vi "BMU参数读取-Auto.vi"(7 "Socket":dbl, 8 "CAN端口":u16(ring), 9 "设备索引号":u16(ring), 10 "CAN卡类型":u32(ring)=21, 11 "从板号":u8=1) -> (3 "成功?":bool)   [LabVIEW 2013] (continued)
          event "读配置文件": Value Change {
            n3737 = event-data() -> ("NewVal"=w5416:bool)  [unwired: 6 out]
            n3738 = case shown="真" w5416 {
              tunnel: w5420 -> [w5422 w5427]
              tunnel: [w5422 w5426] -> w5419
              tunnel: w5418 -> [w5421 w5425]
              tunnel: [w5421 w5424] -> w5417
              frame False {
              }
              frame True {
                n3739 = Enqueue Element(queue=w5427, element="读配置文件", error in (no error)=w5425) -> (queue out=w5426:refnum<queue>, error out=w5424:errorcluster)  [unwired: 2 out]
                n3740 = call <vilib>:"Set Busy.vi"() -> ()  [unwired: 4 in, 8 out]
              }
            }
          }
          event "保存主板参数": Value Change {
            n3741 = event-data() -> ("NewVal"=w5428:bool)  [unwired: 6 out]
            n3742 = case shown="真" w5428 {
              tunnel: w5432 -> [w5434 w5439]
              tunnel: [w5434 w5438] -> w5431
              tunnel: w5430 -> [w5433 w5437]
              tunnel: [w5433 w5436] -> w5429
              frame False {
              }
              frame True {
                n3743 = Enqueue Element(queue=w5439, element="写配置文件", error in (no error)=w5437) -> (queue out=w5438:refnum<queue>, error out=w5436:errorcluster)  [unwired: 2 out]
              }
            }
          }
          event "继电器全开": Value Change {
            n3744 = event-data() -> ("NewVal"=w5440:bool)  [unwired: 6 out]
            n3745 = case shown="真" w5440 {
              tunnel: w5440 -> [_ w5443]
              frame False {
              }
              frame True {
                n3746 = stacked-sequence {
                  tunnel: w5443 -> [_ w5453 _]
                  frame #0 {
                    w5444 = FALSE ("清BUFF")
                    n3747 = local write "正级继电器"(w5444) -> ()
                    n3748 = local write "负级继电器"(w5444) -> ()
                    n3749 = local write "充电继电器"(w5444) -> ()
                    n3750 = local write "加热继电器"(w5444) -> ()
                    n3751 = local write "风机继电器"(w5444) -> ()
                    n3752 = local write "预充电继电器"(w5444) -> ()
                    n3753 = local write "继电器超时处理"(FALSE ("继电器超时处理")) -> ()
                    n3754 = local write "主从选择"(enum32{"主板", "从板"}."主板" ("主从选择")) -> ()
                    n3755 = local write "清BUFF"(FALSE ("清BUFF")) -> ()
                  }
                  frame #1 {
                    n3756 = case shown="真" w5453 {
                      selector: w5453 -> [_ w5468]
                      frame False {
                      }
                      frame True {
                        w5464 = 256.0 ("y")
                        w5455 = u32 1 ("命令序号")
                        w5454 = u8 192 ("命令")
                        n3757 = local read "动作保持时间"() -> (w5465:dbl)
                        n3758 = Quotient & Remainder(x=w5465, y=w5464) -> (x-y*floor(x/y)=w5457:dbl, floor(x/y)=w5461:dbl)
                        n3759 = Quotient & Remainder(x=w5461, y=w5464) -> (x-y*floor(x/y)=w5458:dbl, floor(x/y)=w5462:dbl)
                        n3760 = Quotient & Remainder(x=w5462, y=w5464) -> (x-y*floor(x/y)=w5459:dbl, floor(x/y)=w5463:dbl)
                        n3761 = local read "设备索引号"() -> (w5472:u16)
                        n3762 = local read "CAN卡类型"() -> (w5473:u32)
                        n3763 = local read "CAN端口"() -> (w5471:u16)
                        n3764 = Boolean To (0,1)(Boolean=w5468) -> (0, 1=w5466:i16)
                        n3765 = Quotient & Remainder(x=w5463, y=w5464) -> (x-y*floor(x/y)=w5460:dbl)  [unwired: 1 out]
                        n3766 = Build Array(i16 170 ("元素"), w5466, w5460, w5459, w5458, w5457, 0.0 ("元素")) -> (w5469:dbl[])
                        n3767 = call "多帧发送机制(EV05).vi"("can卡类型"=w5473, "设备索引号"=w5472, "CAN端口"=w5471, "命令"=w5454, "板号"=u8 0, "命令序号"=w5455, "输入数据"=w5469) -> ()  [unwired: 2 in, 11 out]
                        n3768 = local write "命令序号"(w5455) -> ()
                        n3769 = local write "命令"(w5454) -> ()
                      }
                    }
                    n3770 = local write "控制1"(TRUE ("控制1")) -> ()
                    n3771 = local write "写?"(FALSE ("写?")) -> ()
                    n3772 = local write "消除"(TRUE ("消除")) -> ()
                    n3773 = global write "EV05全局变量1.vi" "流控帧 2"(TRUE ("流控帧 2")) -> ()
                    n3774 = global write "EV05全局变量1.vi" "流控帧"(FALSE ("流控帧")) -> ()
                  }
                  frame #2 {
                    n3775 = flat-sequence {
                      tunnel: [w5475] -> w5474
                      tunnel: w5474 -> [w5482]
                      frame #0 {
                        n3776 = while {
                          tunnel: [w5476] -> w5475
                          i -> [w5480]
                          stop <- w5477 stop-if-true
                          n3777 = local read "继电器超时处理"() -> (w5476:bool)
                          n3778 = Greater Or Equal?(x=w5480, y=20) -> (x >= y?=w5478:bool)
                          n3779 = Wait Until Next ms Multiple(millisecond multiple=u32 100 ("毫秒倍数")) -> ()  [unwired: 1 out]
                          n3780 = Or(x=w5476, y=w5478) -> (x .or. y?=w5477:bool)
                        }
                      }
                      frame #1 {
                        n3781 = case shown="真" w5482 {
                          frame False {
                            n3782 = One Button Dialog(message="继电器处理超时" ("消息"), button name ("OK")="是" ("按钮名称（“确定”）")) -> ()  [unwired: 1 out]
                          }
                          frame True {
                            w5485 = TRUE ("清BUFF")
                            n3783 = local write "正级继电器"(w5485) -> ()
                            n3784 = local write "负级继电器"(w5485) -> ()
                            n3785 = local write "充电继电器"(w5485) -> ()
                            n3786 = local write "加热继电器"(w5485) -> ()
                            n3787 = local write "风机继电器"(w5485) -> ()
                            n3788 = local write "预充电继电器"(w5485) -> ()
                          }
                        }
                      }
                    }
                  }
                }
              }
            }
          }
          event "继电器全关": Value Change {
            n3789 = event-data() -> ("NewVal"=w5486:bool)  [unwired: 6 out]
            n3790 = case shown="真" w5486 {
              tunnel: w5486 -> [_ w5489]
              frame False {
              }
              frame True {
                n3791 = stacked-sequence {
                  tunnel: w5489 -> [_ w5499 _]
                  frame #0 {
                    w5490 = TRUE ("清BUFF")
                    n3792 = local write "正级继电器"(w5490) -> ()
                    n3793 = local write "负级继电器"(w5490) -> ()
                    n3794 = local write "充电继电器"(w5490) -> ()
                    n3795 = local write "加热继电器"(w5490) -> ()
                    n3796 = local write "风机继电器"(w5490) -> ()
                    n3797 = local write "预充电继电器"(w5490) -> ()
                    n3798 = local write "继电器超时处理"(FALSE ("继电器超时处理")) -> ()
                    n3799 = local write "主从选择"(enum32{"主板", "从板"}."主板" ("主从选择")) -> ()
                    n3800 = global write "EV05全局变量1.vi" "流控帧"(FALSE ("流控帧")) -> ()
                    n3801 = local write "清BUFF"(FALSE ("清BUFF")) -> ()
                  }
                  frame #1 {
                    n3802 = case shown="真" w5499 {
                      selector: w5499 -> [_ w5514]
                      frame False {
                      }
                      frame True {
                        w5510 = 256.0 ("y")
                        w5501 = u32 1 ("命令序号")
                        w5500 = u8 192 ("命令")
                        n3803 = local read "动作保持时间"() -> (w5511:dbl)
                        n3804 = Quotient & Remainder(x=w5511, y=w5510) -> (x-y*floor(x/y)=w5503:dbl, floor(x/y)=w5507:dbl)
                        n3805 = Quotient & Remainder(x=w5507, y=w5510) -> (x-y*floor(x/y)=w5504:dbl, floor(x/y)=w5508:dbl)
                        n3806 = Quotient & Remainder(x=w5508, y=w5510) -> (x-y*floor(x/y)=w5505:dbl, floor(x/y)=w5509:dbl)
                        n3807 = local read "设备索引号"() -> (w5518:u16)
                        n3808 = local read "CAN卡类型"() -> (w5519:u32)
                        n3809 = local read "CAN端口"() -> (w5517:u16)
                        n3810 = Boolean To (0,1)(Boolean=w5514) -> (0, 1=w5512:i16)
                        n3811 = Quotient & Remainder(x=w5509, y=w5510) -> (x-y*floor(x/y)=w5506:dbl)  [unwired: 1 out]
                        n3812 = Build Array(i16 85 ("元素"), w5512, w5506, w5505, w5504, w5503, 0.0 ("元素")) -> (w5515:dbl[])
                        n3813 = call "多帧发送机制(EV05).vi"("can卡类型"=w5519, "设备索引号"=w5518, "CAN端口"=w5517, "命令"=w5500, "板号"=u8 0, "命令序号"=w5501, "输入数据"=w5515) -> ()  [unwired: 2 in, 11 out]
                        n3814 = local write "命令序号"(w5501) -> ()
                        n3815 = local write "命令"(w5500) -> ()
                      }
                    }
                    n3816 = local write "控制1"(TRUE ("控制1")) -> ()
                    n3817 = local write "写?"(FALSE ("写?")) -> ()
                    n3818 = local write "消除"(TRUE ("消除")) -> ()
                    n3819 = global write "EV05全局变量1.vi" "流控帧 2"(TRUE ("流控帧 2")) -> ()
                  }
                  frame #2 {
                    n3820 = flat-sequence {
                      tunnel: [w5521] -> w5520
                      tunnel: w5520 -> [w5528]
                      frame #0 {
                        n3821 = while {
                          tunnel: [w5522] -> w5521
                          i -> [w5526]
                          stop <- w5523 stop-if-true
                          n3822 = local read "继电器超时处理"() -> (w5522:bool)
                          n3823 = Greater Or Equal?(x=w5526, y=20) -> (x >= y?=w5524:bool)
                          n3824 = Wait Until Next ms Multiple(millisecond multiple=u32 100 ("毫秒倍数")) -> ()  [unwired: 1 out]
                          n3825 = Or(x=w5522, y=w5524) -> (x .or. y?=w5523:bool)
                        }
                      }
                      frame #1 {
                        n3826 = case shown="真" w5528 {
                          frame False {
                            n3827 = One Button Dialog(message="继电器处理超时" ("消息"), button name ("OK")="是" ("按钮名称（“确定”）")) -> ()  [unwired: 1 out]
                          }
                          frame True {
                            w5531 = FALSE ("清BUFF")
                            n3828 = local write "正级继电器"(w5531) -> ()
                            n3829 = local write "负级继电器"(w5531) -> ()
                            n3830 = local write "充电继电器"(w5531) -> ()
                            n3831 = local write "加热继电器"(w5531) -> ()
                            n3832 = local write "风机继电器"(w5531) -> ()
                            n3833 = local write "预充电继电器"(w5531) -> ()
                          }
                        }
                      }
                    }
                  }
                }
              }
            }
          }
          event "控制按键全为开": Value Change {
            n3834 = event-data() -> ("NewVal"=w5532:bool)  [unwired: 6 out]
            n3835 = case shown="真" w5532 {
              frame False {
              }
              frame True {
                w5533 = TRUE ("正级继电器")
                n3836 = local write "加热继电器(从)"(w5533) -> ()
                n3837 = local write "风机继电器(从)"(w5533) -> ()
                n3838 = local write "DO1 2"(w5533) -> ()
                n3839 = local write "DO1"(w5533) -> ()
                n3840 = local write "DO2"(w5533) -> ()
                n3841 = local write "正级继电器"(w5533) -> ()
                n3842 = local write "负级继电器"(w5533) -> ()
                n3843 = local write "加热继电器"(w5533) -> ()
                n3844 = local write "预充电继电器"(w5533) -> ()
                n3845 = local write "充电继电器"(w5533) -> ()
                n3846 = local write "风机继电器"(w5533) -> ()
              }
            }
          }
          event "控制按键全为关": Value Change {
            n3847 = event-data() -> ("NewVal"=w5534:bool)  [unwired: 6 out]
            n3848 = case shown="真" w5534 {
              frame False {
              }
              frame True {
                w5535 = FALSE ("正级继电器")
                n3849 = local write "加热继电器(从)"(w5535) -> ()
                n3850 = local write "风机继电器(从)"(w5535) -> ()
                n3851 = local write "DO1 2"(w5535) -> ()
                n3852 = local write "DO1"(w5535) -> ()
                n3853 = local write "DO2"(w5535) -> ()
                n3854 = local write "正级继电器"(w5535) -> ()
                n3855 = local write "负级继电器"(w5535) -> ()
                n3856 = local write "加热继电器"(w5535) -> ()
                n3857 = local write "预充电继电器"(w5535) -> ()
                n3858 = local write "充电继电器"(w5535) -> ()
                n3859 = local write "风机继电器"(w5535) -> ()
              }
            }
          }
          event "正级继电器": Value Change {
            n3860 = event-data() -> ("NewVal"=w5536:bool)  [unwired: 6 out]
            n3861 = stacked-sequence {
              tunnel: w5536 -> [_ w5549 _]
              frame #0 {
                w5539 = FALSE ("清BUFF")
                n3862 = local write "继电器超时处理"(FALSE ("继电器超时处理")) -> ()
                n3863 = local write "主从选择"(enum32{"主板", "从板"}."主板" ("主从选择")) -> ()
                n3864 = local write "正级继电器 12"(w5539) -> ()
                n3865 = local write "清BUFF"(w5539) -> ()
              }
              frame #1 {
                n3866 = case shown="假" w5549 {
                  selector: w5549 -> [w5564 w5584]
                  tunnel: [w5563 w5583] -> w5548
                  tunnel: [w5551 w5571] -> w5543
                  frame False {
                    w5559 = 256.0 ("y")
                    w5551 = u32 1 ("命令序号")
                    w5563 = u8 192 ("命令")
                    n3867 = local read "动作保持时间"() -> (w5560:dbl)
                    n3868 = Quotient & Remainder(x=w5560, y=w5559) -> (x-y*floor(x/y)=w5552:dbl, floor(x/y)=w5556:dbl)
                    n3869 = Quotient & Remainder(x=w5556, y=w5559) -> (x-y*floor(x/y)=w5553:dbl, floor(x/y)=w5557:dbl)
                    n3870 = Quotient & Remainder(x=w5557, y=w5559) -> (x-y*floor(x/y)=w5554:dbl, floor(x/y)=w5558:dbl)
                    n3871 = local read "设备索引号"() -> (w5568:u16)
                    n3872 = local read "CAN卡类型"() -> (w5569:u32)
                    n3873 = local read "CAN端口"() -> (w5567:u16)
                    n3874 = Boolean To (0,1)(Boolean=w5564) -> (0, 1=w5561:i16)
                    n3875 = Quotient & Remainder(x=w5558, y=w5559) -> (x-y*floor(x/y)=w5555:dbl)  [unwired: 1 out]
                    n3876 = Build Array(i16 1 ("元素"), w5561, w5555, w5554, w5553, w5552, 0.0 ("元素")) -> (w5565:dbl[])
                    n3877 = call "多帧发送机制(EV05).vi"("can卡类型"=w5569, "设备索引号"=w5568, "CAN端口"=w5567, "命令"=w5563, "板号"=u8 0, "命令序号"=w5551, "输入数据"=w5565) -> ()  [unwired: 2 in, 11 out]
                  }
                  frame True {
                    w5579 = 256.0 ("y")
                    w5571 = u32 1 ("命令序号")
                    w5583 = u8 192 ("命令")
                    n3878 = local read "动作保持时间"() -> (w5580:dbl)
                    n3879 = Quotient & Remainder(x=w5580, y=w5579) -> (x-y*floor(x/y)=w5572:dbl, floor(x/y)=w5576:dbl)
                    n3880 = Quotient & Remainder(x=w5576, y=w5579) -> (x-y*floor(x/y)=w5573:dbl, floor(x/y)=w5577:dbl)
                    n3881 = Quotient & Remainder(x=w5577, y=w5579) -> (x-y*floor(x/y)=w5574:dbl, floor(x/y)=w5578:dbl)
                    n3882 = local read "设备索引号"() -> (w5588:u16)
                    n3883 = local read "CAN卡类型"() -> (w5589:u32)
                    n3884 = local read "CAN端口"() -> (w5587:u16)
                    n3885 = Boolean To (0,1)(Boolean=w5584) -> (0, 1=w5581:i16)
                    n3886 = Quotient & Remainder(x=w5578, y=w5579) -> (x-y*floor(x/y)=w5575:dbl)  [unwired: 1 out]
                    n3887 = Build Array(i16 1 ("元素"), w5581, w5575, w5574, w5573, w5572, 0.0 ("元素")) -> (w5585:dbl[])
                    n3888 = call "多帧发送机制(EV05).vi"("can卡类型"=w5589, "设备索引号"=w5588, "CAN端口"=w5587, "命令"=w5583, "板号"=u8 0, "命令序号"=w5571, "输入数据"=w5585) -> ()  [unwired: 2 in, 11 out]
                  }
                }
                n3889 = local write "命令序号"(w5543) -> ()
                n3890 = local write "命令"(w5548) -> ()
                n3891 = local write "控制1"(TRUE ("控制1")) -> ()
                n3892 = local write "写?"(FALSE ("写?")) -> ()
                n3893 = global write "EV05全局变量1.vi" "流控帧"(FALSE ("流控帧")) -> ()
                n3894 = local write "消除"(TRUE ("消除")) -> ()
                n3895 = global write "EV05全局变量1.vi" "流控帧 2"(TRUE ("流控帧 2")) -> ()
              }
              frame #2 {
                n3896 = flat-sequence {
                  tunnel: [w5591] -> w5590
                  tunnel: w5590 -> [w5598]
                  frame #0 {
                    n3897 = while {
                      tunnel: [w5592] -> w5591
                      i -> [w5596]
                      stop <- w5593 stop-if-true
                      n3898 = local read "继电器超时处理"() -> (w5592:bool)
                      n3899 = Greater Or Equal?(x=w5596, y=20) -> (x >= y?=w5594:bool)
                      n3900 = Wait Until Next ms Multiple(millisecond multiple=u32 100 ("毫秒倍数")) -> ()  [unwired: 1 out]
                      n3901 = Or(x=w5592, y=w5594) -> (x .or. y?=w5593:bool)
                    }
                  }
                  frame #1 {
                    n3902 = case shown="假" w5598 {
                      frame False {
                        n3903 = local read "正级继电器"() -> (w5600:bool)
                        n3904 = Not(x=w5600) -> (.not. x?=w5599:bool)
                        n3905 = local write "正级继电器"(w5599) -> ()
                        n3906 = One Button Dialog(message="继电器处理超时" ("消息"), button name ("OK")="是" ("按钮名称（“确定”）")) -> ()  [unwired: 1 out]
                      }
                      frame True {
                      }
                    }
                  }
                }
              }
            }
          }
          event "负级继电器": Value Change {
            n3907 = event-data() -> ("NewVal"=w5603:bool)  [unwired: 6 out]
            n3908 = stacked-sequence {
              tunnel: w5603 -> [_ w5616 _]
              frame #0 {
                w5606 = FALSE ("继电器超时处理")
                n3909 = local write "继电器超时处理"(w5606) -> ()
                n3910 = local write "正级继电器 2"(w5606) -> ()
                n3911 = local write "主从选择"(enum32{"主板", "从板"}."主板" ("主从选择")) -> ()
              }
              frame #1 {
                n3912 = case shown="假" w5616 {
                  selector: w5616 -> [w5630 w5650]
                  tunnel: [w5629 w5649] -> w5615
                  tunnel: [w5618 w5638] -> w5610
                  frame False {
                    w5626 = 256.0 ("y")
                    w5618 = u32 1 ("命令序号")
                    w5629 = u8 192 ("命令")
                    n3913 = local read "动作保持时间"() -> (w5627:dbl)
                    n3914 = Quotient & Remainder(x=w5627, y=w5626) -> (x-y*floor(x/y)=w5619:dbl, floor(x/y)=w5623:dbl)
                    n3915 = Quotient & Remainder(x=w5623, y=w5626) -> (x-y*floor(x/y)=w5620:dbl, floor(x/y)=w5624:dbl)
                    n3916 = Quotient & Remainder(x=w5624, y=w5626) -> (x-y*floor(x/y)=w5621:dbl, floor(x/y)=w5625:dbl)
                    n3917 = Quotient & Remainder(x=w5625, y=w5626) -> (x-y*floor(x/y)=w5622:dbl)  [unwired: 1 out]
                    n3918 = Boolean To (0,1)(Boolean=w5630) -> (0, 1=w5628:i16)
                    n3919 = local read "设备索引号"() -> (w5635:u16)
                    n3920 = local read "CAN卡类型"() -> (w5636:u32)
                    n3921 = local read "CAN端口"() -> (w5634:u16)
                    n3922 = Build Array(i16 2 ("元素"), w5628, w5622, w5621, w5620, w5619, 0.0 ("元素")) -> (w5632:dbl[])
                    n3923 = call "多帧发送机制(EV05).vi"("can卡类型"=w5636, "设备索引号"=w5635, "CAN端口"=w5634, "命令"=w5629, "板号"=u8 0, "命令序号"=w5618, "输入数据"=w5632) -> ()  [unwired: 2 in, 11 out]
                  }
                  frame True {
                    w5646 = 256.0 ("y")
                    w5638 = u32 1 ("命令序号")
                    w5649 = u8 192 ("命令")
                    n3924 = local read "动作保持时间"() -> (w5647:dbl)
                    n3925 = Quotient & Remainder(x=w5647, y=w5646) -> (x-y*floor(x/y)=w5639:dbl, floor(x/y)=w5643:dbl)
                    n3926 = Quotient & Remainder(x=w5643, y=w5646) -> (x-y*floor(x/y)=w5640:dbl, floor(x/y)=w5644:dbl)
                    n3927 = Quotient & Remainder(x=w5644, y=w5646) -> (x-y*floor(x/y)=w5641:dbl, floor(x/y)=w5645:dbl)
                    n3928 = Quotient & Remainder(x=w5645, y=w5646) -> (x-y*floor(x/y)=w5642:dbl)  [unwired: 1 out]
                    n3929 = Boolean To (0,1)(Boolean=w5650) -> (0, 1=w5648:i16)
                    n3930 = local read "设备索引号"() -> (w5655:u16)
                    n3931 = local read "CAN卡类型"() -> (w5656:u32)
                    n3932 = local read "CAN端口"() -> (w5654:u16)
                    n3933 = Build Array(i16 2 ("元素"), w5648, w5642, w5641, w5640, w5639, 0.0 ("元素")) -> (w5652:dbl[])
                    n3934 = call "多帧发送机制(EV05).vi"("can卡类型"=w5656, "设备索引号"=w5655, "CAN端口"=w5654, "命令"=w5649, "板号"=u8 0, "命令序号"=w5638, "输入数据"=w5652) -> ()  [unwired: 2 in, 11 out]
                  }
                }
                n3935 = local write "命令"(w5615) -> ()
                n3936 = local write "命令序号"(w5610) -> ()
                n3937 = local write "清BUFF"(FALSE ("清BUFF")) -> ()
                n3938 = global write "EV05全局变量1.vi" "流控帧"(FALSE ("流控帧")) -> ()
                n3939 = local write "控制1"(TRUE ("控制1")) -> ()
                n3940 = global write "EV05全局变量1.vi" "流控帧 2"(TRUE ("流控帧 2")) -> ()
                n3941 = local write "写?"(FALSE ("写?")) -> ()
                n3942 = local write "消除"(TRUE ("消除")) -> ()
              }
              frame #2 {
                n3943 = flat-sequence {
                  tunnel: [w5658] -> w5657
                  tunnel: w5657 -> [w5665]
                  frame #0 {
                    n3944 = while {
                      tunnel: [w5659] -> w5658
                      i -> [w5663]
                      stop <- w5660 stop-if-true
                      n3945 = local read "继电器超时处理"() -> (w5659:bool)
                      n3946 = Greater Or Equal?(x=w5663, y=20) -> (x >= y?=w5661:bool)
                      n3947 = Wait Until Next ms Multiple(millisecond multiple=u32 100 ("毫秒倍数")) -> ()  [unwired: 1 out]
                      n3948 = Or(x=w5659, y=w5661) -> (x .or. y?=w5660:bool)
                    }
                  }
                  frame #1 {
                    n3949 = case shown="假" w5665 {
                      frame False {
                        n3950 = local read "负级继电器"() -> (w5666:bool)
                        n3951 = Not(x=w5666) -> (.not. x?=w5667:bool)
                        n3952 = local write "负级继电器"(w5667) -> ()
                        n3953 = One Button Dialog(message="继电器处理超时" ("消息"), button name ("OK")="是" ("按钮名称（“确定”）")) -> ()  [unwired: 1 out]
                      }
                      frame True {
                      }
                    }
                  }
                }
              }
            }
          }
          event "预充电继电器": Value Change {
            n3954 = event-data() -> ("NewVal"=w5670:bool)  [unwired: 6 out]
            n3955 = stacked-sequence {
              tunnel: w5670 -> [_ w5683 _]
              frame #0 {
                w5674 = FALSE ("继电器超时处理")
                n3956 = local write "继电器超时处理"(w5674) -> ()
                n3957 = local write "正级继电器 3"(w5674) -> ()
                n3958 = global write "EV05全局变量1.vi" "流控帧"(FALSE ("流控帧")) -> ()
                n3959 = local write "主从选择"(enum32{"主板", "从板"}."主板" ("主从选择")) -> ()
              }
              frame #1 {
                n3960 = case shown="假" w5683 {
                  selector: w5683 -> [w5697 w5717]
                  tunnel: [w5696 w5716] -> w5682
                  tunnel: [w5685 w5705] -> w5677
                  frame False {
                    w5693 = 256.0 ("y")
                    w5685 = u32 1 ("命令序号")
                    w5696 = u8 192 ("命令")
                    n3961 = local read "动作保持时间"() -> (w5694:dbl)
                    n3962 = Quotient & Remainder(x=w5694, y=w5693) -> (x-y*floor(x/y)=w5686:dbl, floor(x/y)=w5690:dbl)
                    n3963 = Quotient & Remainder(x=w5690, y=w5693) -> (x-y*floor(x/y)=w5687:dbl, floor(x/y)=w5691:dbl)
                    n3964 = Quotient & Remainder(x=w5691, y=w5693) -> (x-y*floor(x/y)=w5688:dbl, floor(x/y)=w5692:dbl)
                    n3965 = Quotient & Remainder(x=w5692, y=w5693) -> (x-y*floor(x/y)=w5689:dbl)  [unwired: 1 out]
                    n3966 = Boolean To (0,1)(Boolean=w5697) -> (0, 1=w5695:i16)
                    n3967 = local read "设备索引号"() -> (w5702:u16)
                    n3968 = local read "CAN卡类型"() -> (w5703:u32)
                    n3969 = local read "CAN端口"() -> (w5701:u16)
                    n3970 = Build Array(i16 3 ("元素"), w5695, w5689, w5688, w5687, w5686, 0.0 ("元素")) -> (w5699:dbl[])
                    n3971 = call "多帧发送机制(EV05).vi"("can卡类型"=w5703, "设备索引号"=w5702, "CAN端口"=w5701, "命令"=w5696, "板号"=u8 0, "命令序号"=w5685, "输入数据"=w5699) -> ()  [unwired: 2 in, 11 out]
                  }
                  frame True {
                    w5713 = 256.0 ("y")
                    w5705 = u32 1 ("命令序号")
                    w5716 = u8 192 ("命令")
                    n3972 = local read "动作保持时间"() -> (w5714:dbl)
                    n3973 = Quotient & Remainder(x=w5714, y=w5713) -> (x-y*floor(x/y)=w5706:dbl, floor(x/y)=w5710:dbl)
                    n3974 = Quotient & Remainder(x=w5710, y=w5713) -> (x-y*floor(x/y)=w5707:dbl, floor(x/y)=w5711:dbl)
                    n3975 = Quotient & Remainder(x=w5711, y=w5713) -> (x-y*floor(x/y)=w5708:dbl, floor(x/y)=w5712:dbl)
                    n3976 = Quotient & Remainder(x=w5712, y=w5713) -> (x-y*floor(x/y)=w5709:dbl)  [unwired: 1 out]
                    n3977 = Boolean To (0,1)(Boolean=w5717) -> (0, 1=w5715:i16)
                    n3978 = local read "设备索引号"() -> (w5722:u16)
                    n3979 = local read "CAN卡类型"() -> (w5723:u32)
                    n3980 = local read "CAN端口"() -> (w5721:u16)
                    n3981 = Build Array(i16 3 ("元素"), w5715, w5709, w5708, w5707, w5706, 0.0 ("元素")) -> (w5719:dbl[])
                    n3982 = call "多帧发送机制(EV05).vi"("can卡类型"=w5723, "设备索引号"=w5722, "CAN端口"=w5721, "命令"=w5716, "板号"=u8 0, "命令序号"=w5705, "输入数据"=w5719) -> ()  [unwired: 2 in, 11 out]
                  }
                }
                n3983 = local write "命令序号"(w5677) -> ()
                n3984 = local write "清BUFF"(FALSE ("清BUFF")) -> ()
                n3985 = local write "控制1"(TRUE ("控制1")) -> ()
                n3986 = global write "EV05全局变量1.vi" "流控帧 2"(TRUE ("流控帧 2")) -> ()
                n3987 = local write "消除"(TRUE ("消除")) -> ()
                n3988 = local write "命令"(w5682) -> ()
                n3989 = local write "写?"(FALSE ("写?")) -> ()
              }
              frame #2 {
                n3990 = flat-sequence {
                  tunnel: [w5725] -> w5724
                  tunnel: w5724 -> [w5732]
                  frame #0 {
                    n3991 = while {
                      tunnel: [w5726] -> w5725
                      i -> [w5730]
                      stop <- w5727 stop-if-true
                      n3992 = local read "继电器超时处理"() -> (w5726:bool)
                      n3993 = Greater Or Equal?(x=w5730, y=20) -> (x >= y?=w5728:bool)
                      n3994 = Wait Until Next ms Multiple(millisecond multiple=u32 100 ("毫秒倍数")) -> ()  [unwired: 1 out]
                      n3995 = Or(x=w5726, y=w5728) -> (x .or. y?=w5727:bool)
                    }
                  }
                  frame #1 {
                    n3996 = case shown="假" w5732 {
                      frame False {
                        n3997 = local read "预充电继电器"() -> (w5733:bool)
                        n3998 = Not(x=w5733) -> (.not. x?=w5734:bool)
                        n3999 = local write "预充电继电器"(w5734) -> ()
                        n4000 = One Button Dialog(message="继电器处理超时" ("消息"), button name ("OK")="是" ("按钮名称（“确定”）")) -> ()  [unwired: 1 out]
                      }
                      frame True {
                      }
                    }
                  }
                }
              }
            }
          }
          event "加热继电器": Value Change {
            n4001 = event-data() -> ("NewVal"=w5737:bool)  [unwired: 6 out]
            n4002 = stacked-sequence {
              tunnel: w5737 -> [_ w5750 _]
              frame #0 {
                w5741 = FALSE ("继电器超时处理")
                n4003 = local write "继电器超时处理"(w5741) -> ()
                n4004 = local write "正级继电器 5"(w5741) -> ()
                n4005 = global write "EV05全局变量1.vi" "流控帧"(FALSE ("流控帧")) -> ()
                n4006 = local write "主从选择"(enum32{"主板", "从板"}."主板" ("主从选择")) -> ()
              }
              frame #1 {
                n4007 = case shown="假" w5750 {
                  selector: w5750 -> [w5764 w5784]
                  tunnel: [w5763 w5783] -> w5749
                  tunnel: [w5752 w5772] -> w5744
                  frame False {
                    w5760 = 256.0 ("y")
                    w5752 = u32 1 ("命令序号")
                    w5763 = u8 192 ("命令")
                    n4008 = local read "动作保持时间"() -> (w5761:dbl)
                    n4009 = Quotient & Remainder(x=w5761, y=w5760) -> (x-y*floor(x/y)=w5753:dbl, floor(x/y)=w5757:dbl)
                    n4010 = Quotient & Remainder(x=w5757, y=w5760) -> (x-y*floor(x/y)=w5754:dbl, floor(x/y)=w5758:dbl)
                    n4011 = Quotient & Remainder(x=w5758, y=w5760) -> (x-y*floor(x/y)=w5755:dbl, floor(x/y)=w5759:dbl)
                    n4012 = Quotient & Remainder(x=w5759, y=w5760) -> (x-y*floor(x/y)=w5756:dbl)  [unwired: 1 out]
                    n4013 = Boolean To (0,1)(Boolean=w5764) -> (0, 1=w5762:i16)
                    n4014 = local read "设备索引号"() -> (w5769:u16)
                    n4015 = local read "CAN卡类型"() -> (w5770:u32)
                    n4016 = local read "CAN端口"() -> (w5768:u16)
                    n4017 = Build Array(i16 4 ("元素"), w5762, w5756, w5755, w5754, w5753, 0.0 ("元素")) -> (w5766:dbl[])
                    n4018 = call "多帧发送机制(EV05).vi"("can卡类型"=w5770, "设备索引号"=w5769, "CAN端口"=w5768, "命令"=w5763, "板号"=u8 0, "命令序号"=w5752, "输入数据"=w5766) -> ()  [unwired: 2 in, 11 out]
                  }
                  frame True {
                    w5780 = 256.0 ("y")
                    w5772 = u32 1 ("命令序号")
                    w5783 = u8 192 ("命令")
                    n4019 = local read "动作保持时间"() -> (w5781:dbl)
                    n4020 = Quotient & Remainder(x=w5781, y=w5780) -> (x-y*floor(x/y)=w5773:dbl, floor(x/y)=w5777:dbl)
                    n4021 = Quotient & Remainder(x=w5777, y=w5780) -> (x-y*floor(x/y)=w5774:dbl, floor(x/y)=w5778:dbl)
                    n4022 = Quotient & Remainder(x=w5778, y=w5780) -> (x-y*floor(x/y)=w5775:dbl, floor(x/y)=w5779:dbl)
                    n4023 = Quotient & Remainder(x=w5779, y=w5780) -> (x-y*floor(x/y)=w5776:dbl)  [unwired: 1 out]
                    n4024 = Boolean To (0,1)(Boolean=w5784) -> (0, 1=w5782:i16)
                    n4025 = local read "设备索引号"() -> (w5789:u16)
                    n4026 = local read "CAN卡类型"() -> (w5790:u32)
                    n4027 = local read "CAN端口"() -> (w5788:u16)
                    n4028 = Build Array(i16 4 ("元素"), w5782, w5776, w5775, w5774, w5773, 0.0 ("元素")) -> (w5786:dbl[])
                    n4029 = call "多帧发送机制(EV05).vi"("can卡类型"=w5790, "设备索引号"=w5789, "CAN端口"=w5788, "命令"=w5783, "板号"=u8 0, "命令序号"=w5772, "输入数据"=w5786) -> ()  [unwired: 2 in, 11 out]
                  }
                }
                n4030 = local write "命令序号"(w5744) -> ()
                n4031 = local write "清BUFF"(FALSE ("清BUFF")) -> ()
                n4032 = local write "命令"(w5749) -> ()
                n4033 = local write "控制1"(TRUE ("控制1")) -> ()
                n4034 = local write "写?"(FALSE ("写?")) -> ()
                n4035 = global write "EV05全局变量1.vi" "流控帧 2"(TRUE ("流控帧 2")) -> ()
                n4036 = local write "消除"(TRUE ("消除")) -> ()
              }
              frame #2 {
                n4037 = flat-sequence {
                  tunnel: [w5792] -> w5791
                  tunnel: w5791 -> [w5799]
                  frame #0 {
                    n4038 = while {
                      tunnel: [w5793] -> w5792
                      i -> [w5797]
                      stop <- w5794 stop-if-true
                      n4039 = local read "继电器超时处理"() -> (w5793:bool)
                      n4040 = Greater Or Equal?(x=w5797, y=20) -> (x >= y?=w5795:bool)
                      n4041 = Wait Until Next ms Multiple(millisecond multiple=u32 100 ("毫秒倍数")) -> ()  [unwired: 1 out]
                      n4042 = Or(x=w5793, y=w5795) -> (x .or. y?=w5794:bool)
                    }
                  }
                  frame #1 {
                    n4043 = case shown="假" w5799 {
                      frame False {
                        n4044 = local read "加热继电器"() -> (w5800:bool)
                        n4045 = Not(x=w5800) -> (.not. x?=w5801:bool)
                        n4046 = local write "加热继电器"(w5801) -> ()
                        n4047 = One Button Dialog(message="继电器处理超时" ("消息"), button name ("OK")="是" ("按钮名称（“确定”）")) -> ()  [unwired: 1 out]
                      }
                      frame True {
                      }
                    }
                  }
                }
              }
            }
          }
          event "充电继电器": Value Change {
            n4048 = event-data() -> ("NewVal"=w5804:bool)  [unwired: 6 out]
            n4049 = stacked-sequence {
              tunnel: w5804 -> [_ w5817 _]
              frame #0 {
                w5808 = FALSE ("继电器超时处理")
                n4050 = local write "主从选择"(enum32{"主板", "从板"}."主板" ("主从选择")) -> ()
                n4051 = global write "EV05全局变量1.vi" "流控帧"(FALSE ("流控帧")) -> ()
                n4052 = local write "继电器超时处理"(w5808) -> ()
                n4053 = local write "正级继电器 4"(w5808) -> ()
              }
              frame #1 {
                n4054 = case shown="假" w5817 {
                  selector: w5817 -> [w5831 w5851]
                  tunnel: [w5830 w5850] -> w5816
                  tunnel: [w5819 w5839] -> w5811
                  frame False {
                    w5827 = 256.0 ("y")
                    w5819 = u32 1 ("命令序号")
                    w5830 = u8 192 ("命令")
                    n4055 = local read "动作保持时间"() -> (w5828:dbl)
                    n4056 = Quotient & Remainder(x=w5828, y=w5827) -> (x-y*floor(x/y)=w5820:dbl, floor(x/y)=w5824:dbl)
                    n4057 = Quotient & Remainder(x=w5824, y=w5827) -> (x-y*floor(x/y)=w5821:dbl, floor(x/y)=w5825:dbl)
                    n4058 = Quotient & Remainder(x=w5825, y=w5827) -> (x-y*floor(x/y)=w5822:dbl, floor(x/y)=w5826:dbl)
                    n4059 = Quotient & Remainder(x=w5826, y=w5827) -> (x-y*floor(x/y)=w5823:dbl)  [unwired: 1 out]
                    n4060 = Boolean To (0,1)(Boolean=w5831) -> (0, 1=w5829:i16)
                    n4061 = local read "设备索引号"() -> (w5836:u16)
                    n4062 = local read "CAN卡类型"() -> (w5837:u32)
                    n4063 = local read "CAN端口"() -> (w5835:u16)
                    n4064 = Build Array(i16 5 ("元素"), w5829, w5823, w5822, w5821, w5820, 0.0 ("元素")) -> (w5833:dbl[])
                    n4065 = call "多帧发送机制(EV05).vi"("can卡类型"=w5837, "设备索引号"=w5836, "CAN端口"=w5835, "命令"=w5830, "板号"=u8 0, "命令序号"=w5819, "输入数据"=w5833) -> ()  [unwired: 2 in, 11 out]
                  }
                  frame True {
                    w5847 = 256.0 ("y")
                    w5839 = u32 1 ("命令序号")
                    w5850 = u8 192 ("命令")
                    n4066 = local read "动作保持时间"() -> (w5848:dbl)
                    n4067 = Quotient & Remainder(x=w5848, y=w5847) -> (x-y*floor(x/y)=w5840:dbl, floor(x/y)=w5844:dbl)
                    n4068 = Quotient & Remainder(x=w5844, y=w5847) -> (x-y*floor(x/y)=w5841:dbl, floor(x/y)=w5845:dbl)
                    n4069 = Quotient & Remainder(x=w5845, y=w5847) -> (x-y*floor(x/y)=w5842:dbl, floor(x/y)=w5846:dbl)
                    n4070 = Quotient & Remainder(x=w5846, y=w5847) -> (x-y*floor(x/y)=w5843:dbl)  [unwired: 1 out]
                    n4071 = Boolean To (0,1)(Boolean=w5851) -> (0, 1=w5849:i16)
                    n4072 = local read "设备索引号"() -> (w5856:u16)
                    n4073 = local read "CAN卡类型"() -> (w5857:u32)
                    n4074 = local read "CAN端口"() -> (w5855:u16)
                    n4075 = Build Array(i16 5 ("元素"), w5849, w5843, w5842, w5841, w5840, 0.0 ("元素")) -> (w5853:dbl[])
                    n4076 = call "多帧发送机制(EV05).vi"("can卡类型"=w5857, "设备索引号"=w5856, "CAN端口"=w5855, "命令"=w5850, "板号"=u8 0, "命令序号"=w5839, "输入数据"=w5853) -> ()  [unwired: 2 in, 11 out]
                  }
                }
                n4077 = local write "命令序号"(w5811) -> ()
                n4078 = local write "命令"(w5816) -> ()
                n4079 = local write "清BUFF"(FALSE ("清BUFF")) -> ()
                n4080 = local write "控制1"(TRUE ("控制1")) -> ()
                n4081 = global write "EV05全局变量1.vi" "流控帧 2"(TRUE ("流控帧 2")) -> ()
                n4082 = local write "写?"(FALSE ("写?")) -> ()
                n4083 = local write "消除"(TRUE ("消除")) -> ()
              }
              frame #2 {
                n4084 = flat-sequence {
                  tunnel: [w5859] -> w5858
                  tunnel: w5858 -> [w5866]
                  frame #0 {
                    n4085 = while {
                      tunnel: [w5860] -> w5859
                      i -> [w5864]
                      stop <- w5861 stop-if-true
                      n4086 = local read "继电器超时处理"() -> (w5860:bool)
                      n4087 = Greater Or Equal?(x=w5864, y=20) -> (x >= y?=w5862:bool)
                      n4088 = Wait Until Next ms Multiple(millisecond multiple=u32 100 ("毫秒倍数")) -> ()  [unwired: 1 out]
                      n4089 = Or(x=w5860, y=w5862) -> (x .or. y?=w5861:bool)
                    }
                  }
                  frame #1 {
                    n4090 = case shown="假" w5866 {
                      frame False {
                        n4091 = local read "充电继电器"() -> (w5867:bool)
                        n4092 = Not(x=w5867) -> (.not. x?=w5868:bool)
                        n4093 = local write "充电继电器"(w5868) -> ()
                        n4094 = One Button Dialog(message="继电器处理超时" ("消息"), button name ("OK")="是" ("按钮名称（“确定”）")) -> ()  [unwired: 1 out]
                      }
                      frame True {
                      }
                    }
                  }
                }
              }
            }
          }
          event "风机继电器": Value Change {
            n4095 = event-data() -> ("NewVal"=w5871:bool)  [unwired: 6 out]
            n4096 = stacked-sequence {
              tunnel: w5871 -> [_ w5884 _]
              frame #0 {
                w5875 = FALSE ("继电器超时处理")
                n4097 = local write "继电器超时处理"(w5875) -> ()
                n4098 = local write "正级继电器 6"(w5875) -> ()
                n4099 = global write "EV05全局变量1.vi" "流控帧"(FALSE ("流控帧")) -> ()
                n4100 = local write "主从选择"(enum32{"主板", "从板"}."主板" ("主从选择")) -> ()
              }
              frame #1 {
                n4101 = case shown="真" w5884 {
                  selector: w5884 -> [w5898 w5918]
                  tunnel: [w5897 w5917] -> w5883
                  tunnel: [w5886 w5906] -> w5878
                  frame True {
                    w5894 = 256.0 ("y")
                    w5886 = u32 1 ("命令序号")
                    w5897 = u8 192 ("命令")
                    n4102 = local read "动作保持时间"() -> (w5895:dbl)
                    n4103 = Quotient & Remainder(x=w5895, y=w5894) -> (x-y*floor(x/y)=w5887:dbl, floor(x/y)=w5891:dbl)
                    n4104 = Quotient & Remainder(x=w5891, y=w5894) -> (x-y*floor(x/y)=w5888:dbl, floor(x/y)=w5892:dbl)
                    n4105 = Quotient & Remainder(x=w5892, y=w5894) -> (x-y*floor(x/y)=w5889:dbl, floor(x/y)=w5893:dbl)
                    n4106 = Boolean To (0,1)(Boolean=w5898) -> (0, 1=w5896:i16)
                    n4107 = local read "设备索引号"() -> (w5903:u16)
                    n4108 = local read "CAN卡类型"() -> (w5904:u32)
                    n4109 = Quotient & Remainder(x=w5893, y=w5894) -> (x-y*floor(x/y)=w5890:dbl)  [unwired: 1 out]
                    n4110 = local read "CAN端口"() -> (w5902:u16)
                    n4111 = Build Array(i16 6 ("元素"), w5896, w5890, w5889, w5888, w5887, 0.0 ("元素")) -> (w5900:dbl[])
                    n4112 = call "多帧发送机制(EV05).vi"("can卡类型"=w5904, "设备索引号"=w5903, "CAN端口"=w5902, "命令"=w5897, "板号"=u8 0, "命令序号"=w5886, "输入数据"=w5900) -> ()  [unwired: 2 in, 11 out]
                  }
                  frame False {
                    w5914 = 256.0 ("y")
                    w5906 = u32 1 ("命令序号")
                    w5917 = u8 192 ("命令")
                    n4113 = local read "动作保持时间"() -> (w5915:dbl)
                    n4114 = Quotient & Remainder(x=w5915, y=w5914) -> (x-y*floor(x/y)=w5907:dbl, floor(x/y)=w5911:dbl)
                    n4115 = Quotient & Remainder(x=w5911, y=w5914) -> (x-y*floor(x/y)=w5908:dbl, floor(x/y)=w5912:dbl)
                    n4116 = Quotient & Remainder(x=w5912, y=w5914) -> (x-y*floor(x/y)=w5909:dbl, floor(x/y)=w5913:dbl)
                    n4117 = Boolean To (0,1)(Boolean=w5918) -> (0, 1=w5916:i16)
                    n4118 = local read "设备索引号"() -> (w5923:u16)
                    n4119 = local read "CAN卡类型"() -> (w5924:u32)
                    n4120 = Quotient & Remainder(x=w5913, y=w5914) -> (x-y*floor(x/y)=w5910:dbl)  [unwired: 1 out]
                    n4121 = local read "CAN端口"() -> (w5922:u16)
                    n4122 = Build Array(i16 6 ("元素"), w5916, w5910, w5909, w5908, w5907, 0.0 ("元素")) -> (w5920:dbl[])
                    n4123 = call "多帧发送机制(EV05).vi"("can卡类型"=w5924, "设备索引号"=w5923, "CAN端口"=w5922, "命令"=w5917, "板号"=u8 0, "命令序号"=w5906, "输入数据"=w5920) -> ()  [unwired: 2 in, 11 out]
                  }
                }
                n4124 = local write "命令序号"(w5878) -> ()
                n4125 = local write "命令"(w5883) -> ()
                n4126 = local write "清BUFF"(FALSE ("清BUFF")) -> ()
                n4127 = local write "控制1"(TRUE ("控制1")) -> ()
                n4128 = global write "EV05全局变量1.vi" "流控帧 2"(TRUE ("流控帧 2")) -> ()
                n4129 = local write "写?"(FALSE ("写?")) -> ()
                n4130 = local write "消除"(TRUE ("消除")) -> ()
              }
              frame #2 {
                n4131 = flat-sequence {
                  tunnel: [w5926] -> w5925
                  tunnel: w5925 -> [w5933]
                  frame #0 {
                    n4132 = while {
                      tunnel: [w5927] -> w5926
                      i -> [w5931]
                      stop <- w5928 stop-if-true
                      n4133 = local read "继电器超时处理"() -> (w5927:bool)
                      n4134 = Greater Or Equal?(x=w5931, y=20) -> (x >= y?=w5929:bool)
                      n4135 = Wait Until Next ms Multiple(millisecond multiple=u32 100 ("毫秒倍数")) -> ()  [unwired: 1 out]
                      n4136 = Or(x=w5927, y=w5929) -> (x .or. y?=w5928:bool)
                    }
                  }
                  frame #1 {
                    n4137 = case shown="假" w5933 {
                      frame False {
                        n4138 = local read "风机继电器"() -> (w5934:bool)
                        n4139 = Not(x=w5934) -> (.not. x?=w5935:bool)
                        n4140 = local write "风机继电器"(w5935) -> ()
                        n4141 = One Button Dialog(message="继电器处理超时" ("消息"), button name ("OK")="是" ("按钮名称（“确定”）")) -> ()  [unwired: 1 out]
                      }
                      frame True {
                      }
                    }
                  }
                }
              }
            }
          }
          event "加热继电器(从)": Value Change {
            n4142 = event-data() -> ("NewVal"=w5938:bool)  [unwired: 6 out]
            n4143 = stacked-sequence {
              tunnel: w5938 -> [_ w5952 _]
              frame #0 {
                w5942 = FALSE ("继电器超时处理")
                n4144 = local write "正级继电器 7"(w5942) -> ()
                n4145 = local write "继电器超时处理"(w5942) -> ()
                n4146 = global write "EV05全局变量1.vi" "流控帧"(FALSE ("流控帧")) -> ()
                n4147 = local write "主从选择"(enum32{"主板", "从板"}."从板" ("主从选择")) -> ()
              }
              frame #1 {
                n4148 = case shown="真" w5952 {
                  selector: w5952 -> [w5967 w5987]
                  tunnel: [w5966 w5986] -> w5951
                  tunnel: [w5965 w5985] -> w5945
                  tunnel: [w5954 w5974] -> w5946
                  frame True {
                    w5962 = 256.0 ("y")
                    w5954 = u32 1 ("命令序号")
                    w5966 = u8 192 ("命令")
                    n4149 = local read "动作保持时间"() -> (w5963:dbl)
                    n4150 = Quotient & Remainder(x=w5963, y=w5962) -> (x-y*floor(x/y)=w5955:dbl, floor(x/y)=w5959:dbl)
                    n4151 = Quotient & Remainder(x=w5959, y=w5962) -> (x-y*floor(x/y)=w5956:dbl, floor(x/y)=w5960:dbl)
                    n4152 = Quotient & Remainder(x=w5960, y=w5962) -> (x-y*floor(x/y)=w5957:dbl, floor(x/y)=w5961:dbl)
                    n4153 = Quotient & Remainder(x=w5961, y=w5962) -> (x-y*floor(x/y)=w5958:dbl)  [unwired: 1 out]
                    n4154 = Boolean To (0,1)(Boolean=w5967) -> (0, 1=w5964:i16)
                    n4155 = local read "设备索引号"() -> (w5971:u16)
                    n4156 = local read "CAN卡类型"() -> (w5972:u32)
                    n4157 = local read "从板板号"() -> (w5965:u8)
                    n4158 = local read "CAN端口"() -> (w5970:u16)
                    n4159 = Build Array(i16 7 ("元素"), w5964, w5958, w5957, w5956, w5955, 0.0 ("元素")) -> (w5969:dbl[])
                    n4160 = call "多帧发送机制(EV05).vi"("can卡类型"=w5972, "设备索引号"=w5971, "CAN端口"=w5970, "命令"=w5966, "板号"=w5965, "命令序号"=w5954, "输入数据"=w5969) -> ()  [unwired: 2 in, 11 out]
                  }
                  frame False {
                    w5982 = 256.0 ("y")
                    w5974 = u32 1 ("命令序号")
                    w5986 = u8 192 ("命令")
                    n4161 = local read "动作保持时间"() -> (w5983:dbl)
                    n4162 = Quotient & Remainder(x=w5983, y=w5982) -> (x-y*floor(x/y)=w5975:dbl, floor(x/y)=w5979:dbl)
                    n4163 = Quotient & Remainder(x=w5979, y=w5982) -> (x-y*floor(x/y)=w5976:dbl, floor(x/y)=w5980:dbl)
                    n4164 = Quotient & Remainder(x=w5980, y=w5982) -> (x-y*floor(x/y)=w5977:dbl, floor(x/y)=w5981:dbl)
                    n4165 = Quotient & Remainder(x=w5981, y=w5982) -> (x-y*floor(x/y)=w5978:dbl)  [unwired: 1 out]
                    n4166 = Boolean To (0,1)(Boolean=w5987) -> (0, 1=w5984:i16)
                    n4167 = local read "设备索引号"() -> (w5991:u16)
                    n4168 = local read "CAN卡类型"() -> (w5992:u32)
                    n4169 = local read "从板板号"() -> (w5985:u8)
                    n4170 = local read "CAN端口"() -> (w5990:u16)
                    n4171 = Build Array(i16 7 ("元素"), w5984, w5978, w5977, w5976, w5975, 0.0 ("元素")) -> (w5989:dbl[])
                    n4172 = call "多帧发送机制(EV05).vi"("can卡类型"=w5992, "设备索引号"=w5991, "CAN端口"=w5990, "命令"=w5986, "板号"=w5985, "命令序号"=w5974, "输入数据"=w5989) -> ()  [unwired: 2 in, 11 out]
                  }
                }
                n4173 = local write "从板板号"(w5945) -> ()
                n4174 = local write "命令序号"(w5946) -> ()
                n4175 = local write "命令"(w5951) -> ()
                n4176 = local write "清BUFF"(FALSE ("清BUFF")) -> ()
                n4177 = local write "写?"(FALSE ("写?")) -> ()
                n4178 = local write "控制1"(TRUE ("控制1")) -> ()
                n4179 = global write "EV05全局变量1.vi" "流控帧 2"(TRUE ("流控帧 2")) -> ()
                n4180 = local write "消除"(TRUE ("消除")) -> ()
              }
              frame #2 {
                n4181 = flat-sequence {
                  tunnel: [w5994] -> w5993
                  tunnel: w5993 -> [w6001]
                  frame #0 {
                    n4182 = while {
                      tunnel: [w5995] -> w5994
                      i -> [w5999]
                      stop <- w5996 stop-if-true
                      n4183 = local read "继电器超时处理"() -> (w5995:bool)
                      n4184 = Greater Or Equal?(x=w5999, y=20) -> (x >= y?=w5997:bool)
                      n4185 = Wait Until Next ms Multiple(millisecond multiple=u32 100 ("毫秒倍数")) -> ()  [unwired: 1 out]
                      n4186 = Or(x=w5995, y=w5997) -> (x .or. y?=w5996:bool)
                    }
                  }
                  frame #1 {
                    n4187 = case shown="假" w6001 {
                      frame False {
                        n4188 = local read "加热继电器(从)"() -> (w6003:bool)
                        n4189 = Not(x=w6003) -> (.not. x?=w6002:bool)
                        n4190 = local write "加热继电器(从)"(w6002) -> ()
                        n4191 = One Button Dialog(message="继电器处理超时" ("消息"), button name ("OK")="是" ("按钮名称（“确定”）")) -> ()  [unwired: 1 out]
                      }
                      frame True {
                      }
                    }
                  }
                }
              }
            }
          }
          event "风机继电器(从)": Value Change {
            n4192 = event-data() -> ("NewVal"=w6006:bool)  [unwired: 6 out]
            n4193 = stacked-sequence {
              tunnel: w6006 -> [_ w6020 _]
              frame #0 {
                w6010 = FALSE ("继电器超时处理")
                n4194 = local write "继电器超时处理"(w6010) -> ()
                n4195 = local write "正级继电器 8"(w6010) -> ()
                n4196 = global write "EV05全局变量1.vi" "流控帧"(FALSE ("流控帧")) -> ()
                n4197 = local write "主从选择"(enum32{"主板", "从板"}."从板" ("主从选择")) -> ()
              }
              frame #1 {
                n4198 = case shown="假" w6020 {
                  selector: w6020 -> [w6035 w6055]
                  tunnel: [w6034 w6054] -> w6019
                  tunnel: [w6033 w6053] -> w6013
                  tunnel: [w6022 w6042] -> w6014
                  frame False {
                    w6030 = 256.0 ("y")
                    w6022 = u32 1 ("命令序号")
                    w6034 = u8 192 ("命令")
                    n4199 = local read "动作保持时间"() -> (w6031:dbl)
                    n4200 = Quotient & Remainder(x=w6031, y=w6030) -> (x-y*floor(x/y)=w6023:dbl, floor(x/y)=w6027:dbl)
                    n4201 = Quotient & Remainder(x=w6027, y=w6030) -> (x-y*floor(x/y)=w6024:dbl, floor(x/y)=w6028:dbl)
                    n4202 = Quotient & Remainder(x=w6028, y=w6030) -> (x-y*floor(x/y)=w6025:dbl, floor(x/y)=w6029:dbl)
                    n4203 = Quotient & Remainder(x=w6029, y=w6030) -> (x-y*floor(x/y)=w6026:dbl)  [unwired: 1 out]
                    n4204 = local read "设备索引号"() -> (w6039:u16)
                    n4205 = local read "CAN卡类型"() -> (w6040:u32)
                    n4206 = local read "从板板号"() -> (w6033:u8)
                    n4207 = Boolean To (0,1)(Boolean=w6035) -> (0, 1=w6032:i16)
                    n4208 = local read "CAN端口"() -> (w6038:u16)
                    n4209 = Build Array(i16 8 ("元素"), w6032, w6026, w6025, w6024, w6023, 0.0 ("元素")) -> (w6037:dbl[])
                    n4210 = call "多帧发送机制(EV05).vi"("can卡类型"=w6040, "设备索引号"=w6039, "CAN端口"=w6038, "命令"=w6034, "板号"=w6033, "命令序号"=w6022, "输入数据"=w6037) -> ()  [unwired: 2 in, 11 out]
                  }
                  frame True {
                    w6050 = 256.0 ("y")
                    w6042 = u32 1 ("命令序号")
                    w6054 = u8 192 ("命令")
                    n4211 = local read "动作保持时间"() -> (w6051:dbl)
                    n4212 = Quotient & Remainder(x=w6051, y=w6050) -> (x-y*floor(x/y)=w6043:dbl, floor(x/y)=w6047:dbl)
                    n4213 = Quotient & Remainder(x=w6047, y=w6050) -> (x-y*floor(x/y)=w6044:dbl, floor(x/y)=w6048:dbl)
                    n4214 = Quotient & Remainder(x=w6048, y=w6050) -> (x-y*floor(x/y)=w6045:dbl, floor(x/y)=w6049:dbl)
                    n4215 = Quotient & Remainder(x=w6049, y=w6050) -> (x-y*floor(x/y)=w6046:dbl)  [unwired: 1 out]
                    n4216 = local read "设备索引号"() -> (w6059:u16)
                    n4217 = local read "CAN卡类型"() -> (w6060:u32)
                    n4218 = local read "从板板号"() -> (w6053:u8)
                    n4219 = Boolean To (0,1)(Boolean=w6055) -> (0, 1=w6052:i16)
                    n4220 = local read "CAN端口"() -> (w6058:u16)
                    n4221 = Build Array(i16 8 ("元素"), w6052, w6046, w6045, w6044, w6043, 0.0 ("元素")) -> (w6057:dbl[])
                    n4222 = call "多帧发送机制(EV05).vi"("can卡类型"=w6060, "设备索引号"=w6059, "CAN端口"=w6058, "命令"=w6054, "板号"=w6053, "命令序号"=w6042, "输入数据"=w6057) -> ()  [unwired: 2 in, 11 out]
                  }
                }
                n4223 = local write "从板板号"(w6013) -> ()
                n4224 = local write "清BUFF"(FALSE ("清BUFF")) -> ()
                n4225 = local write "命令序号"(w6014) -> ()
                n4226 = local write "命令"(w6019) -> ()
                n4227 = local write "控制1"(TRUE ("控制1")) -> ()
                n4228 = local write "写?"(FALSE ("写?")) -> ()
                n4229 = local write "消除"(TRUE ("消除")) -> ()
                n4230 = global write "EV05全局变量1.vi" "流控帧 2"(TRUE ("流控帧 2")) -> ()
              }
              frame #2 {
                n4231 = flat-sequence {
                  tunnel: [w6062] -> w6061
                  tunnel: w6061 -> [w6069]
                  frame #0 {
                    n4232 = while {
                      tunnel: [w6063] -> w6062
                      i -> [w6067]
                      stop <- w6064 stop-if-true
                      n4233 = local read "继电器超时处理"() -> (w6063:bool)
                      n4234 = Greater Or Equal?(x=w6067, y=20) -> (x >= y?=w6065:bool)
                      n4235 = Wait Until Next ms Multiple(millisecond multiple=u32 100 ("毫秒倍数")) -> ()  [unwired: 1 out]
                      n4236 = Or(x=w6063, y=w6065) -> (x .or. y?=w6064:bool)
                    }
                  }
                  frame #1 {
                    n4237 = case shown="假" w6069 {
                      frame False {
                        n4238 = local read "风机继电器(从)"() -> (w6071:bool)
                        n4239 = Not(x=w6071) -> (.not. x?=w6070:bool)
                        n4240 = local write "风机继电器(从)"(w6070) -> ()
                        n4241 = One Button Dialog(message="继电器处理超时" ("消息"), button name ("OK")="是" ("按钮名称（“确定”）")) -> ()  [unwired: 1 out]
                      }
                      frame True {
                      }
                    }
                  }
                }
              }
